vi "test 8- syslevelModeCallsChainMode.vi"(8 "error in (no error)":errorcluster, 11 "TestCase in":refnum<class "testcase-SyncMessage.lvclass">) -> (0 "error out":errorcluster, 3 "TestCase out":refnum<class "testcase-SyncMessage.lvclass">)   [LabVIEW 2017, in "testcase-SyncMessage.lvclass"]
uses:
  testcase-SyncMessage.lvclass
  <vilib>/addons/_JKI Toolkits/VI Tester/TestCase.llb/TestCase.lvclass
  src/user.lib/_NEVSTOP/Communicable State Machine(CSM)/Communicable State Machine.lvlib
  C:/Program Files (x86)/National Instruments/LabVIEW 2017/vi.lib/addons/_JKI Toolkits/VI Tester/TestCase.llb/TestCase.lvclass
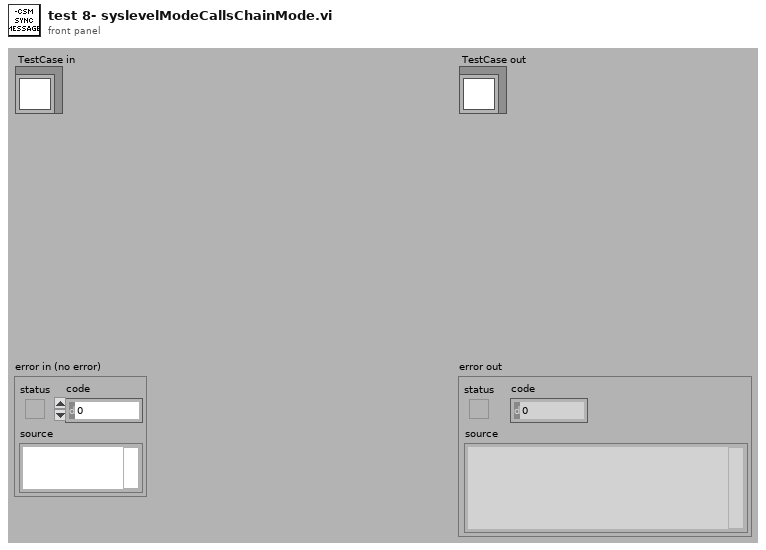
[diagram p1: front panel]
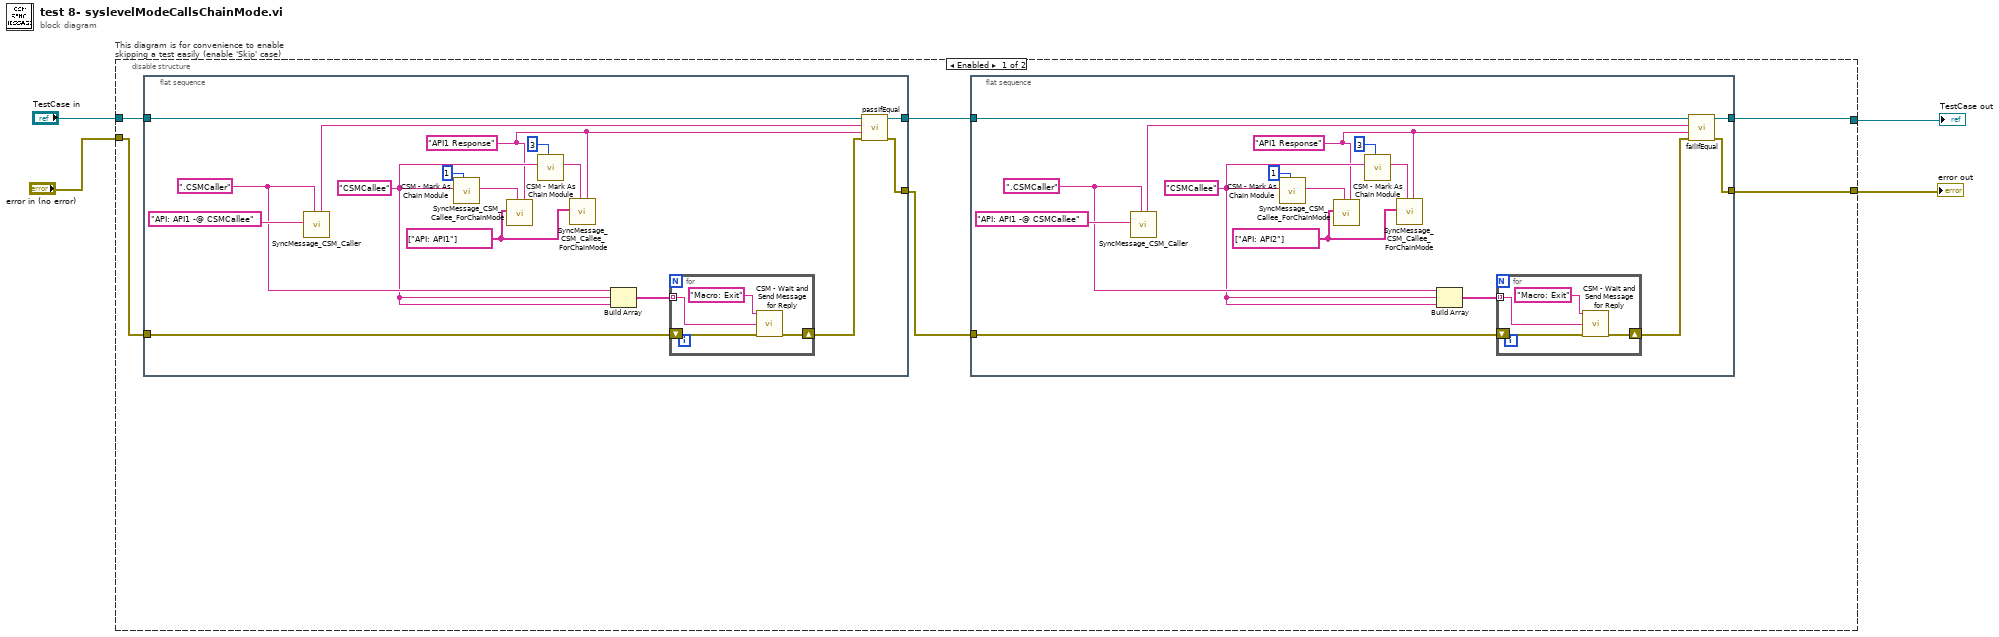
[diagram p0: block diagram]
diagram:
  n1 = disable-structure "This diagram is for convenience to enable skipping a test easily (enable 'Skip' case)" shown="Enabled" {
    disable-tunnel: "TestCase in" -> [w10 w54]
    disable-tunnel: [w8 w52] -> w2
    disable-tunnel: [w6 w53] -> w1
    disable-tunnel: "error in (no error)" -> [w5 w51]
    frame Enabled {
      n2 = flat-sequence {
        tunnel: w10 -> [w46]
        tunnel: [w45] -> w9
        tunnel: [w44] -> w7
        tunnel: w5 -> [w31]
        frame #0 {
          w36 = string[] ["API: API1"] ("Allowed Messages (Empty for All)")
          w35 = "CSMCallee" ("CSMCallee")
          w40 = ".CSMCaller" ("CSMCaller")
          w32 = "API1 Response" ("API response in")
          n3 = call "SyncMessage_CSM_Caller.vi"("Name (\"\" to Use UUID)"=w40, "Intermodule Message in"="API: API1 -@ CSMCallee") -> ("API received Response out"=w42:string)  [unwired: 9 in]
          n4 = call "CSM - Mark As Chain Module.vi"("Order"=1, "CSM Name"=w35) -> ("CSM Name (Marked As Chain)"=w37:string)  [unwired: 8 in]
          n5 = call "SyncMessage_CSM_Callee_ForChainMode.vi"("API response in"=w32, "Name (\"\" to Use UUID)"=w37, "Allowed Messages (Empty for All)"=w36) -> ()  [unwired: 9 in]
          n6 = call "CSM - Mark As Chain Module.vi"("Order"=3, "CSM Name"=w35) -> ("CSM Name (Marked As Chain)"=w33:string)  [unwired: 8 in]
          n7 = call "SyncMessage_CSM_Callee_ForChainMode.vi"("API response in"=w32, "Name (\"\" to Use UUID)"=w33, "Allowed Messages (Empty for All)"=w36) -> ()  [unwired: 9 in]
          n8 = Build Array(w40, w35, w35) -> (w41:string[])
          n9 = for {
            shift-right: [w48] -> w39
            shift-left: w31 -> [w49]
            tunnel: w41 -> [w47] mode=indexing
            n10 = call "CSM - Wait and Send Message for Reply.vi"("State"="Macro: Exit", "Target Module"=w47, "Error In (No Error)"=w49) -> ("error out"=w48:errorcluster)  [unwired: 10 in, 2 out]
          }
          n11 = call-dynamic "passIfEqual.vi"("error in (no error)"=w39, "y"=w32, "x"=w42, "TestCase in"=w46) -> ("error out"=w44:errorcluster, "TestCase out"=w45:refnum<class "testcase-SyncMessage.lvclass">)  [unwired: 6 in]
        }
      }
      n12 = flat-sequence {
        tunnel: w9 -> [w26]
        tunnel: [w25] -> w8
        tunnel: [w24] -> w6
        tunnel: w7 -> [w11]
        frame #0 {
          w16 = string[] ["API: API2"] ("Allowed Messages (Empty for All)")
          w15 = "CSMCallee" ("CSMCallee")
          w20 = ".CSMCaller" ("CSMCaller")
          w12 = "API1 Response" ("API response in")
          n13 = call "SyncMessage_CSM_Caller.vi"("Name (\"\" to Use UUID)"=w20, "Intermodule Message in"="API: API1 -@ CSMCallee") -> ("API received Response out"=w22:string)  [unwired: 9 in]
          n14 = call "CSM - Mark As Chain Module.vi"("Order"=1, "CSM Name"=w15) -> ("CSM Name (Marked As Chain)"=w17:string)  [unwired: 8 in]
          n15 = call "SyncMessage_CSM_Callee_ForChainMode.vi"("API response in"=w12, "Name (\"\" to Use UUID)"=w17, "Allowed Messages (Empty for All)"=w16) -> ()  [unwired: 9 in]
          n16 = call "CSM - Mark As Chain Module.vi"("Order"=3, "CSM Name"=w15) -> ("CSM Name (Marked As Chain)"=w13:string)  [unwired: 8 in]
          n17 = call "SyncMessage_CSM_Callee_ForChainMode.vi"("API response in"=w12, "Name (\"\" to Use UUID)"=w13, "Allowed Messages (Empty for All)"=w16) -> ()  [unwired: 9 in]
          n18 = Build Array(w20, w15, w15) -> (w21:string[])
          n19 = for {
            shift-right: [w28] -> w19
            shift-left: w11 -> [w29]
            tunnel: w21 -> [w27] mode=indexing
            n20 = call "CSM - Wait and Send Message for Reply.vi"("State"="Macro: Exit", "Target Module"=w27, "Error In (No Error)"=w29) -> ("error out"=w28:errorcluster)  [unwired: 10 in, 2 out]
          }
          n21 = call-dynamic "failIfEqual.vi"("error in (no error)"=w19, "y"=w12, "x"=w22, "TestCase in"=w26) -> ("error out"=w24:errorcluster, "TestCase out"=w25:refnum<class "testcase-SyncMessage.lvclass">)  [unwired: 6 in]
        }
      }
    }
    frame Disabled {
      # "skip test result while test is under development"
      n22 = call <vilib>:"skip.vi"("error in (no error)"=w51, "TestCase in"=w54) -> ("error out"=w53:errorcluster, "TestCase out"=w52:refnum<class "testcase-SyncMessage.lvclass">)  [unwired: 8 in]
    }
  }
  "error out" <- w1
  "TestCase out" <- w2
